vi "test_ConfigureBoard.vi"() -> (0 "error out":errorcluster)   [LabVIEW 2020]
uses:
  <instrlib>/AIM GmbH/_AIM 664/_controls/port_configuration.ctl
  <instrlib>/AIM GmbH/_AIM 664/_controls/port_speed.ctl
  <instrlib>/AIM GmbH/_AIM 664/bsp/Fdx Create Session (Generic-Board).vi
  <instrlib>/AIM GmbH/_AIM 664/AIM664LV.lvlib
panel:
  in  "PortSpeed":T1[](array[typedef])=[0, 0] items=["FDX_100MBIT"=0, "FDX_10MBIT"=1, "FDX_1000MBIT"=5, "FDX_AUTO_100MBIT"=2, "FDX_AUTO_10MBIT"=3]
  in  "PortConfig":T2[](array[typedef])=[0, 0] items=["FDX_SINGLE", "FDX_REDUNDANT"]
  out "timed out":bool
  out "good link":bool
  in  "timeout (ms)":u32=10000
  in  "board":u32
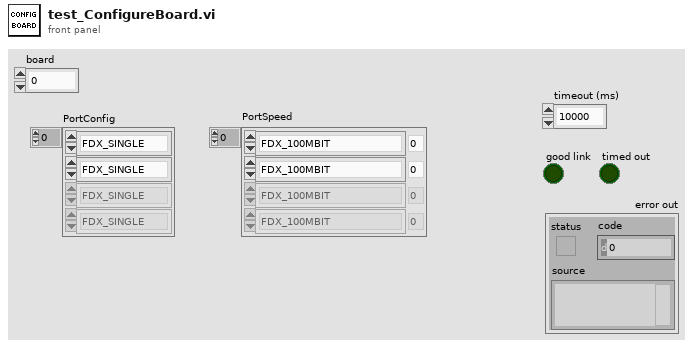
[diagram p1: front panel]
types:
  T1 = typedef "AIM664LV.lvlib/port_speed.ctl" = u32
  T2 = typedef "AIM664LV.lvlib/port_configuration.ctl" = u32
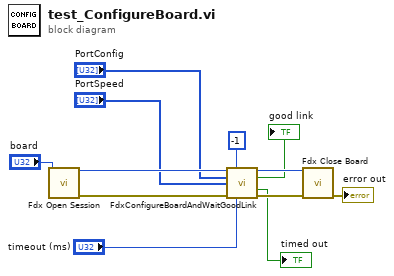
[diagram p0: block diagram]
diagram:
  n1 = call-poly <instrlib>:"Fdx Open Session.vi"("board"="board") -> ("error out"=w6:errorcluster, "InstrumentHandle_board out"=w12:u32)  [unwired: 8 in, 1 out]
  n2 = call <instrlib>:"FdxConfigureBoardAndWaitGoodLink.vi"("InstrumentHandle_board in"=w12, "Port for Goodlink (-1 is all)"=-1, "PortConfig"="PortConfig", "PortSpeed"="PortSpeed", "error in"=w6, "timeout (ms)"="timeout (ms)") -> ("InstrumentHandle_board out"=w10:u32, "good link"=→"good link":bool, "timed out"=→"timed out":bool, "error out"=w9:errorcluster)  [unwired: 6 in]
  n3 = call <instrlib>:"Fdx Close Board.vi"("error in"=w9, "InstrumentHandle_board in"=w10) -> ("error out"=→"error out":errorcluster)  [unwired: 9 in]
